vi "CustomError.vi"(11 "String":string) -> (0 "error out":errorcluster)   [LabVIEW 2017]
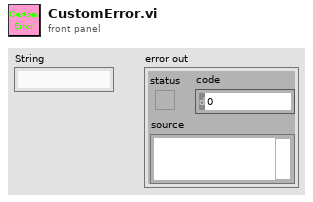
[diagram p1: front panel]
types:
  T1 = cluster{"Status":bool, "Code":u32, "String":string}
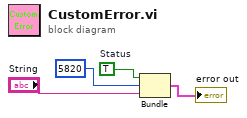
[diagram p0: block diagram]
diagram:
  w3 = TRUE  # Status
  n1 = Bundle("Status"=w3, "Code"=u32 5820, "String"="String") -> (→"error out":T1)  [unwired: 1 in]
